vi "Get Robot Position.vi"(10 "Odometry Data":dbl[](array[numeric]), 11 "Camera Position":T1) -> (1 "Up Direction":cluster{"index":sgl, "index":sgl, "index":sgl}, 2 "Target":cluster{"DBL":dbl, "DBL":dbl, "index":sgl}, 3 "Camera Position":cluster{dbl, dbl, sgl})   [LabVIEW 2017]
uses:
  <vilib>/Utility/miscctls.llb/LV3DPointTypeDef.ctl
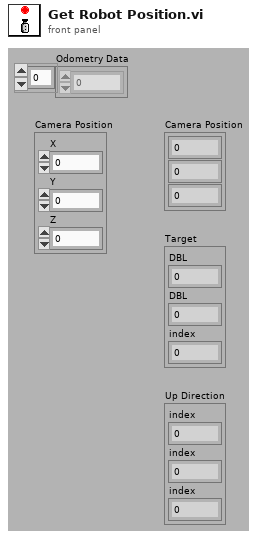
[diagram p1: front panel]
types:
  T1 = typedef "LV3DPointTypeDef.ctl" = cluster{"X":sgl, "Y":sgl, "Z":sgl}
  T2 = cluster{"Numeric":dbl, "Numeric":dbl, "index 2":sgl}
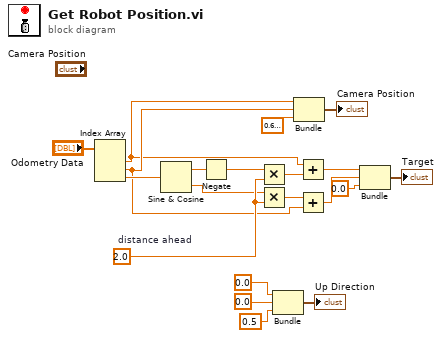
[diagram p0: block diagram]
diagram:
  w9 = sgl 2.0  # distance ahead
  n1 = Index Array(array="Odometry Data") -> (element #1=w1:dbl, element #2=w2:dbl, element #3=w4:dbl)  [unwired: 3 in]
  n2 = Sine & Cosine(0:w4) -> (1:w5:dbl, 2:w6:dbl)
  n3 = Negate(x=w5) -> (-x=w3:dbl)
  n4 = Multiply(x=w3, y=w9) -> (x*y=w11:dbl)
  n5 = Multiply(x=w6, y=w9) -> (x*y=w10:dbl)
  n6 = Bundle("index"=sgl 0.0, "index"=sgl 0.0, "index"=sgl 0.5) -> (→"Up Direction":cluster{"index":sgl, "index":sgl, "index":sgl})  [unwired: 1 in]
  n7 = Bundle("Numeric"=w1, "Numeric"=w2, "index 2"=sgl 0.7) -> (→"Camera Position":T2)  [unwired: 1 in]
  n8 = Add(x=w1, y=w11) -> (x+y=w8:dbl)
  n9 = Add(x=w10, y=w2) -> (x+y=w7:dbl)
  n10 = Bundle(w8, w7, "index"=sgl 0.0) -> (→"Target":cluster{dbl, dbl, "index":sgl})  [unwired: 1 in]
